vi "Database-ActorMain.vi"(0 "FTW Actor Instance Configuration":string="{\n  \"Identity\": \"ActorName\",\n  \"InboxAddress\": \"tcp://127.0.0.1:*\",\n  \"PublisherAddress\": \"tcp://127.0.0.1:*\",\n  \"DebugEnableInboxLogging\": false,\n  \"DebugEnableJobLogging\": false,\n  \"DebugShowPanel\": false\n}", 11 "error in":errorcluster) -> (15 "error out":errorcluster)   [LabVIEW 2013, in "PartCertDatabase-Actor.lvclass"]
uses:
  PartCertDatabase-Actor.lvclass
  ftw-dataflow/Actor/src/Instance/FTW-ActorInstance.lvclass
  ftw-dataflow/Actor/src/Message/Request/FTW-Message-IncomingRequest.lvclass
  PCert-Container/ERP-ConfigPageNewFeather/PCert-ConfigPageNF.lvclass
panel:
  # "Inputs"
  # "Outputs"
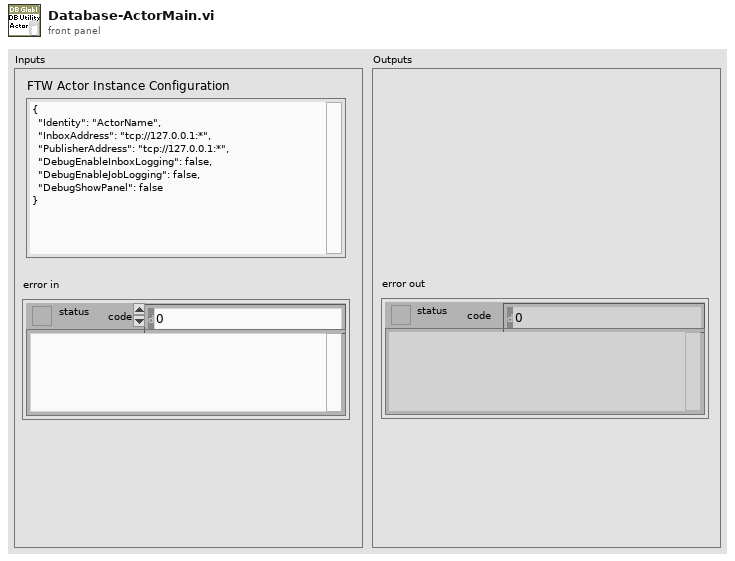
[diagram p1: front panel]
types:
  T1 = cluster{"Incoming Requests":refnum<event-registration>, "Additional Registration Types":refnum<event-registration>}
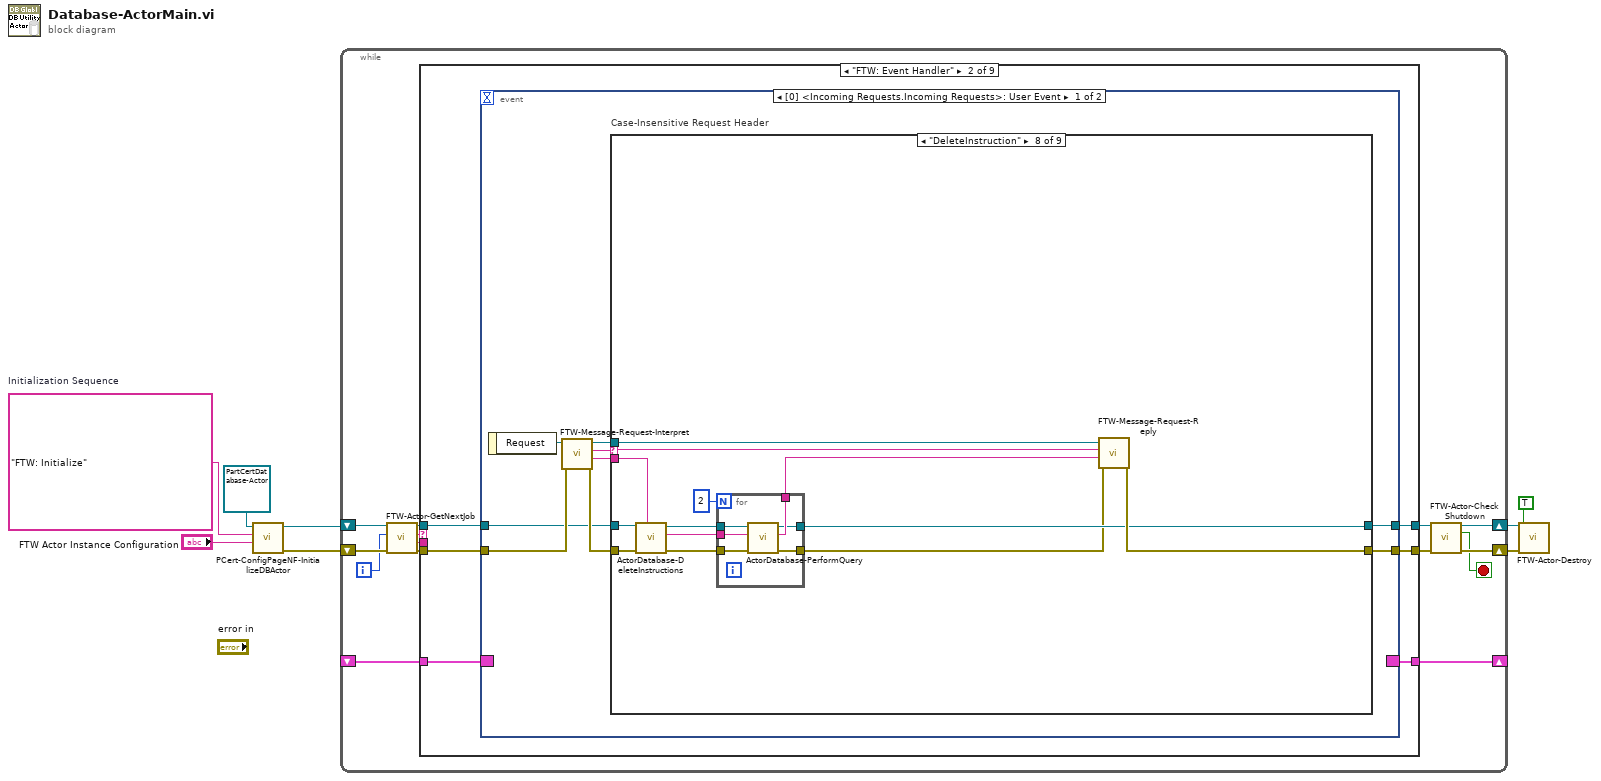
[diagram p0: block diagram]
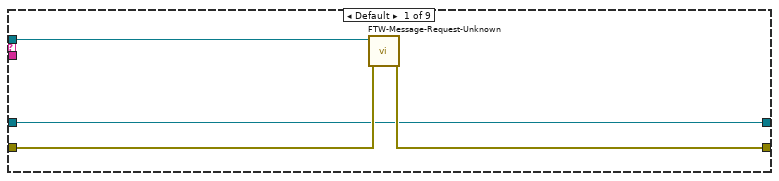
[diagram p3: hidden frame]
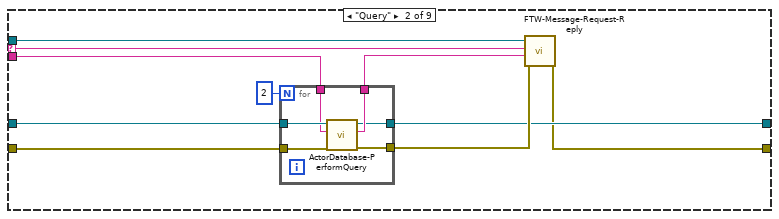
[diagram p4: hidden frame]
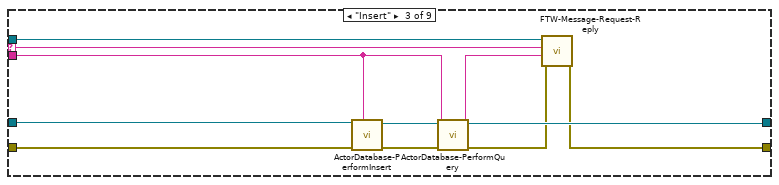
[diagram p5: hidden frame]
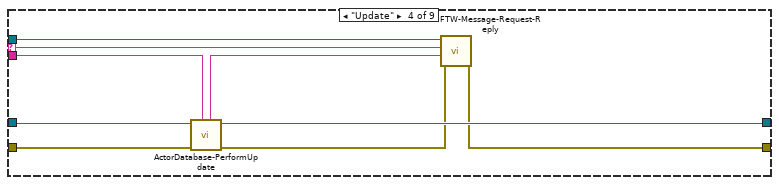
[diagram p6: hidden frame]
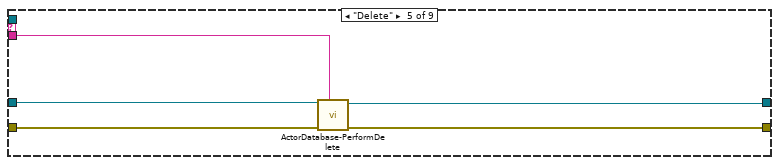
[diagram p7: hidden frame]
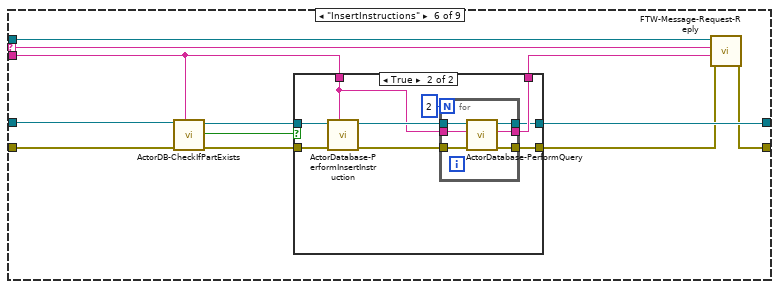
[diagram p8: hidden frame]
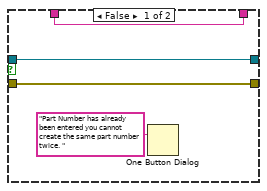
[diagram p9: hidden frame]
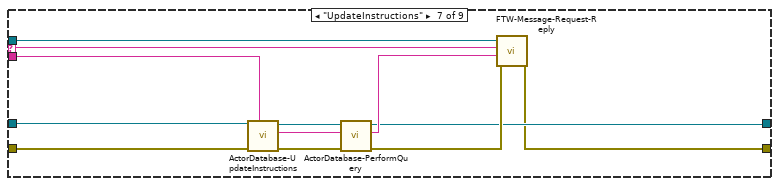
[diagram p10: hidden frame]
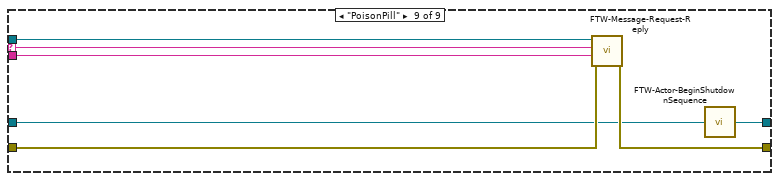
[diagram p11: hidden frame]
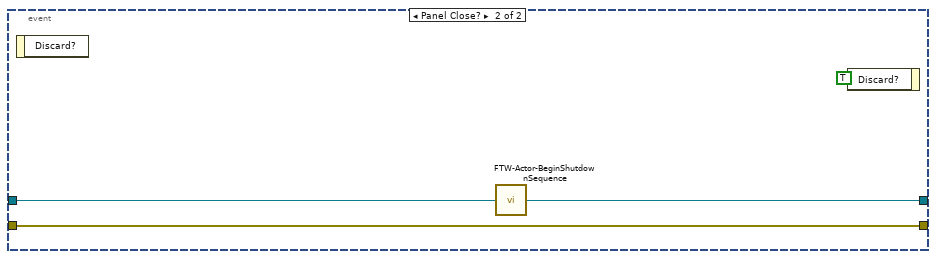
[diagram p12: hidden frame]
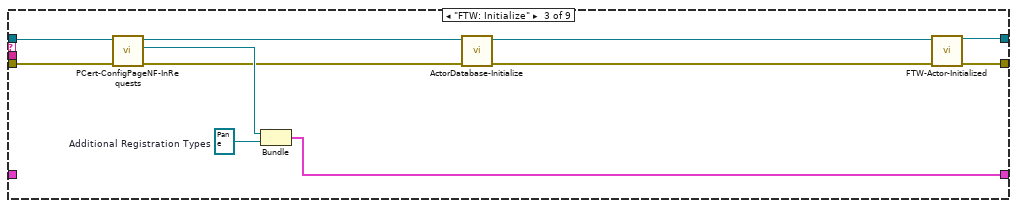
[diagram p13: hidden frame]
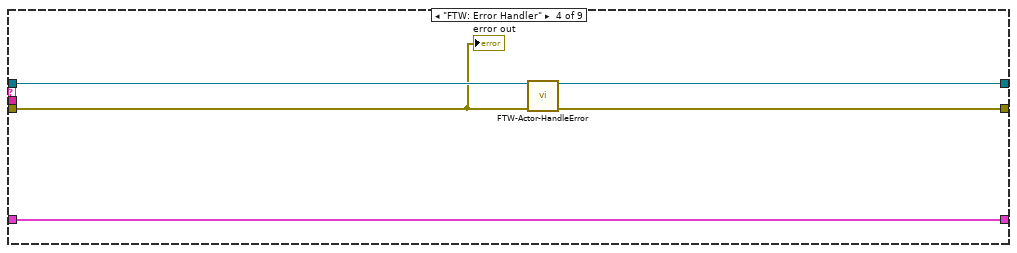
[diagram p14: hidden frame]
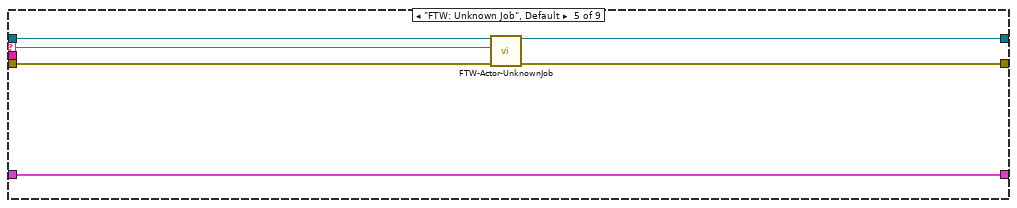
[diagram p15: hidden frame]
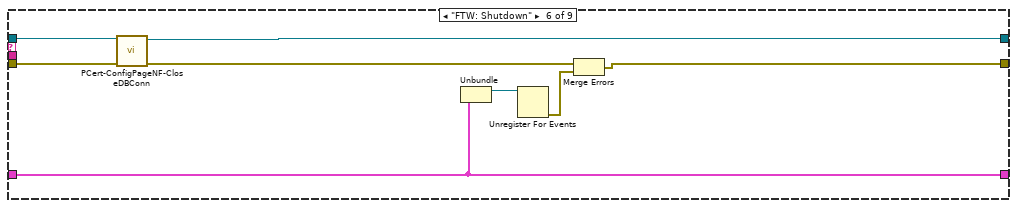
[diagram p16: hidden frame]
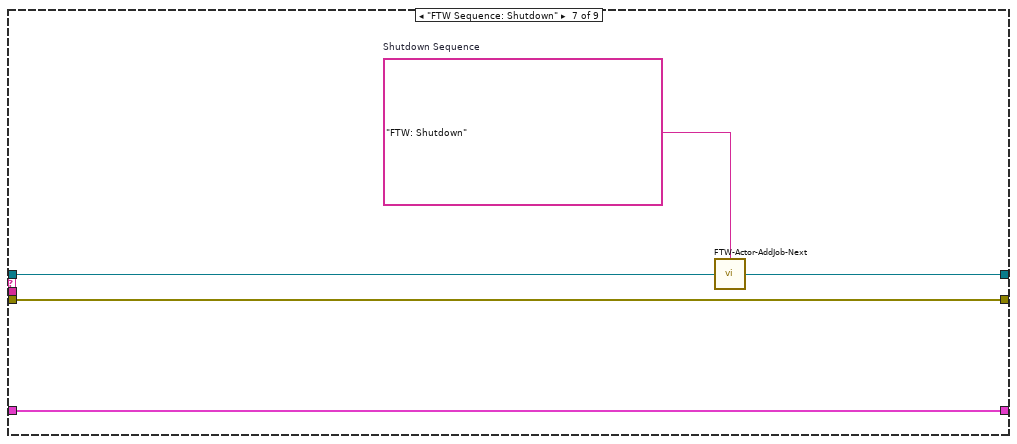
[diagram p17: hidden frame]
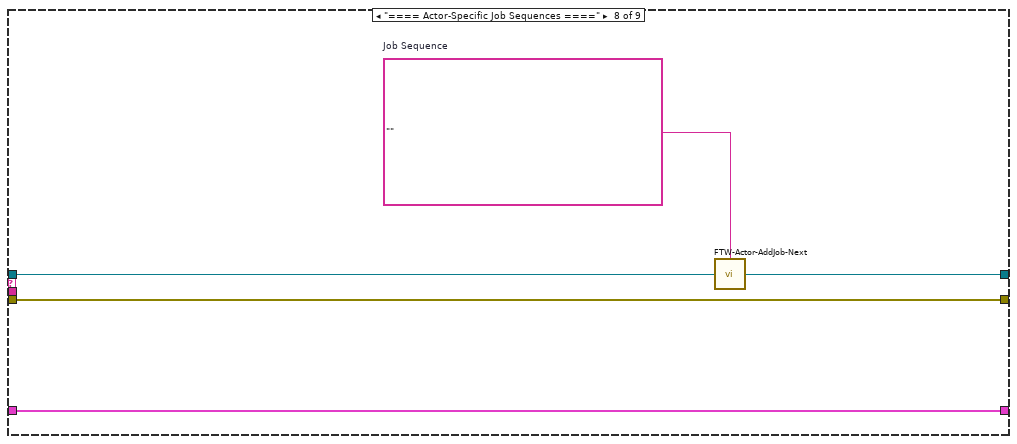
[diagram p18: hidden frame]
diagram:
  w4 = "FTW: Initialize"  # Initialization Sequence
  n1 = call-dynamic "PCert-ConfigPageNF-InitializeDBActor.vi"("FTW Actor Instance Configuration"="FTW Actor Instance Configuration", "Initialization Job Sequence"=w4, "ERP-ConfigPageNF.lvclass"=refnum<class "PartCertDatabase-Actor.lvclass"> refnum ("Database-Actor.lvclass")) -> ("error out"=w6:errorcluster, "ERP-ConfigPageNF out"=w3:refnum<class "PartCertDatabase-Actor.lvclass">)  [unwired: 7 in]
  n2 = while {
    shift-right: [w12] -> w7
    shift-left: w6 -> [w19]
    shift-right: [w9] -> _
    shift-left: _ -> [w22]
    shift-right: [w14] -> w8
    shift-left: w3 -> [w21]
    i -> [w10]
    stop <- w11 stop-if-true
    n3 = call "FTW-Actor-GetNextJob.vi"("error in"=w19, "Jobs Performed"=w10, "FTW Actor Instance"=w21) -> ("error out"=w18:errorcluster, "Job Data"=w16:string, "Job Name"=w17:string, "FTW Actor Instance out"=w20:refnum<class "PartCertDatabase-Actor.lvclass">)  [unwired: 5 in]
    n4 = case shown="\"FTW: Event Handler\"" w17 {
      selector: w17 -> [_ _ _ _ w175 _ _ _ _]
      tunnel: [w24 w31 w164 w171 w178 w186 w192 w197 w201] -> w13
      tunnel: w18 -> [w24 w30 w169 w170 w179 w183 w192 w197 w201]
      tunnel: w22 -> [w25 w26 _ w174 w180 w188 w193 w198 w200]
      tunnel: [w25 w29 w166 w174 w180 w188 w193 w198 w200] -> w9
      tunnel: w16 -> [_ _ _ _ _ _ _ _ _]
      tunnel: [w23 w28 w165 w172 w176 w182 w190 w195 w199] -> w15
      tunnel: w20 -> [w23 w27 w163 w173 w177 w184 w191 w196 w199]
      frame "==== Featherweight Framework Jobs ====" {
      }
      frame "FTW: Event Handler" {
        n5 = event shown="[0] <Incoming Requests.Incoming Requests>: User Event" {
          selector: w26 -> [_ _]
          dyn-events: [_ _] -> w29
          timeout: _ -> [_ _]
          tunnel: [w37 w157] -> w31
          tunnel: w30 -> [w38 w157]
          tunnel: [w36 w155] -> w28
          tunnel: w27 -> [w35 w156]
          event User Event {
            n6 = event-data() -> ("Request"=w39:refnum<class "FTW-Message-IncomingRequest.lvclass">)  [unwired: 1 in]
            n7 = call "FTW-Message-Request-Interpret.vi"("error in"=w38, "FTW Incoming Request"=w39) -> ("error out"=w40:errorcluster, "Request Body"=w33:string, "Request Header"=w34:string, "FTW Incoming Request out"=w32:refnum<class "FTW-Message-IncomingRequest.lvclass">)  [unwired: 6 in]
            n8 = case "Case-Insensitive Request Header" shown="\"DeleteInstruction\"" w34 {
              selector: w34 -> [_ w47 w66 w74 _ w92 w121 w138 w150]
              tunnel: [w43 w46 w63 w72 w83 w94 w118 w137 w151] -> w37
              tunnel: w40 -> [w44 w54 w62 w80 w85 w90 w128 w141 w152]
              tunnel: [w41 w48 w67 w77 w84 w96 w119 w133 w154] -> w36
              tunnel: w35 -> [w41 w53 w61 w79 w82 w91 w127 w140 w148]
              tunnel: w33 -> [_ w52 w69 w78 w81 w89 w124 w135 w149]
              tunnel: w32 -> [w42 w51 w68 w76 _ w93 w122 w139 w153]
              frame Default {
                n9 = call "FTW-Message-Request-Unknown.vi"("error in"=w44, "FTW Incoming Request"=w42) -> ("error out"=w43:errorcluster)  [unwired: 9 in]
              }
              frame "Query" {
                n10 = for {
                  N: 2 -> [_]
                  tunnel: w54 -> [w60]
                  tunnel: w53 -> [w59]
                  tunnel: w52 -> [w58]
                  tunnel: [w57] -> w50
                  tunnel: [w56] -> w49
                  tunnel: [w55] -> w48
                  n11 = call "ActorDatabase-PerformQuery.vi"("error in (no error)"=w60, "Payload from Actor"=w58, "Database-Actor in"=w59) -> ("error out"=w56:errorcluster, "Payload To Actor"=w57:string, "Database-Actor out"=w55:refnum<class "PartCertDatabase-Actor.lvclass">)  [unwired: 6 in]
                }
                n12 = call "FTW-Message-Request-Reply.vi"("error in"=w49, "Response Body"=w50, "Response Header"=w47, "FTW Incoming Request"=w51) -> ("error out"=w46:errorcluster)  [unwired: 6 in, 1 out]
              }
              frame "Insert" {
                n13 = call "ActorDatabase-PerformInsert.vi"("Payload From Actor"=w69, "error in (no error)"=w62, "Database-Actor in"=w61) -> ("error out"=w71:errorcluster, "Database-Actor out"=w70:refnum<class "PartCertDatabase-Actor.lvclass">)  [unwired: 7 in]
                n14 = call "ActorDatabase-PerformQuery.vi"("error in (no error)"=w71, "Payload from Actor"=w69, "Database-Actor in"=w70) -> ("error out"=w64:errorcluster, "Payload To Actor"=w65:string, "Database-Actor out"=w67:refnum<class "PartCertDatabase-Actor.lvclass">)  [unwired: 6 in]
                n15 = call "FTW-Message-Request-Reply.vi"("error in"=w64, "Response Body"=w65, "Response Header"=w66, "FTW Incoming Request"=w68) -> ("error out"=w63:errorcluster)  [unwired: 6 in, 1 out]
              }
              frame "Update" {
                n16 = call "ActorDatabase-PerformUpdate.vi"("Payload From Actor"=w78, "error in (no error)"=w80, "Database-Actor in"=w79) -> ("error out"=w73:errorcluster, "Database-Actor out"=w77:refnum<class "PartCertDatabase-Actor.lvclass">, "Payload to Actor"=w75:string)  [unwired: 6 in]
                n17 = call "FTW-Message-Request-Reply.vi"("error in"=w73, "Response Body"=w75, "Response Header"=w74, "FTW Incoming Request"=w76) -> ("error out"=w72:errorcluster)  [unwired: 6 in, 1 out]
              }
              frame "Delete" {
                n18 = call "ActorDatabase-PerformDelete.vi"("Payload From Actor"=w81, "error in (no error)"=w85, "Database-Actor in"=w82) -> ("error out"=w83:errorcluster, "Database-Actor out"=w84:refnum<class "PartCertDatabase-Actor.lvclass">)  [unwired: 7 in]
              }
              frame "InsertInstructions" {
                n19 = call "ActorDB-CheckIfPartExists.vi"("Request Body"=w89, "error in"=w90, "Database-Actor in"=w91) -> ("error out"=w88:errorcluster, "Part number not found?"=w86:bool, "Database-Actor out"=w87:refnum<class "PartCertDatabase-Actor.lvclass">)  [unwired: 6 in]
                n20 = case shown="True" w86 {
                  tunnel: [w101 w109] -> w97
                  tunnel: [w100 w108] -> w96
                  tunnel: [w99 w107] -> w95
                  tunnel: w89 -> [w101 w106]
                  tunnel: w88 -> [w99 w105]
                  tunnel: w87 -> [w100 w104]
                  frame False {
                    n21 = One Button Dialog(message="Part Number has already been entered you cannot create the same part number twice. ") -> ()  [unwired: 1 in, 1 out]
                  }
                  frame True {
                    n22 = call "ActorDatabase-PerformInsertInstruction.vi"("Payload From Actor"=w106, "error in (no error)"=w105, "Database-Actor in"=w104) -> ("error out"=w102:errorcluster, "Database-Actor out"=w110:refnum<class "PartCertDatabase-Actor.lvclass">)  [unwired: 7 in]
                    n23 = for {
                      N: 2 -> [_]
                      tunnel: w110 -> [w116]
                      tunnel: [w115] -> w109
                      tunnel: [w114] -> w108
                      tunnel: [w113] -> w107
                      tunnel: w106 -> [w112]
                      tunnel: w102 -> [w111]
                      n24 = call "ActorDatabase-PerformQuery.vi"("error in (no error)"=w111, "Payload from Actor"=w112, "Database-Actor in"=w116) -> ("error out"=w113:errorcluster, "Payload To Actor"=w115:string, "Database-Actor out"=w114:refnum<class "PartCertDatabase-Actor.lvclass">)  [unwired: 6 in]
                    }
                  }
                }
                n25 = call "FTW-Message-Request-Reply.vi"("error in"=w95, "Response Body"=w97, "Response Header"=w92, "FTW Incoming Request"=w93) -> ("error out"=w94:errorcluster)  [unwired: 6 in, 1 out]
              }
              frame "UpdateInstructions" {
                n26 = call "ActorDatabase-UpdateInstructions.vi"("Payload From Actor"=w124, "error in (no error)"=w128, "Database-Actor in"=w127) -> ("error out"=w126:errorcluster, "JSON Query"=w117:string, "Database-Actor out"=w125:refnum<class "PartCertDatabase-Actor.lvclass">)  [unwired: 6 in]
                n27 = call "ActorDatabase-PerformQuery.vi"("error in (no error)"=w126, "Payload from Actor"=w117, "Database-Actor in"=w125) -> ("error out"=w120:errorcluster, "Payload To Actor"=w123:string, "Database-Actor out"=w119:refnum<class "PartCertDatabase-Actor.lvclass">)  [unwired: 6 in]
                n28 = call "FTW-Message-Request-Reply.vi"("error in"=w120, "Response Body"=w123, "Response Header"=w121, "FTW Incoming Request"=w122) -> ("error out"=w118:errorcluster)  [unwired: 6 in, 1 out]
              }
              frame "DeleteInstruction" {
                n29 = call "ActorDatabase-DeleteInstructions.vi"("Payload From Actor"=w135, "error in (no error)"=w141, "Database-Actor in"=w140) -> ("error out"=w130:errorcluster, "New Payload"=w131:string, "Database-Actor out"=w136:refnum<class "PartCertDatabase-Actor.lvclass">)  [unwired: 6 in]
                n30 = for {
                  N: 2 -> [_]
                  tunnel: w136 -> [w147]
                  tunnel: [w146] -> w134
                  tunnel: [w145] -> w133
                  tunnel: [w144] -> w132
                  tunnel: w131 -> [w143]
                  tunnel: w130 -> [w142]
                  n31 = call "ActorDatabase-PerformQuery.vi"("error in (no error)"=w142, "Payload from Actor"=w143, "Database-Actor in"=w147) -> ("error out"=w144:errorcluster, "Payload To Actor"=w146:string, "Database-Actor out"=w145:refnum<class "PartCertDatabase-Actor.lvclass">)  [unwired: 6 in]
                }
                n32 = call "FTW-Message-Request-Reply.vi"("error in"=w132, "Response Body"=w134, "Response Header"=w138, "FTW Incoming Request"=w139) -> ("error out"=w137:errorcluster)  [unwired: 6 in, 1 out]
              }
              frame "PoisonPill" {
                n33 = call "FTW-Message-Request-Reply.vi"("error in"=w152, "Response Body"=w149, "Response Header"=w150, "FTW Incoming Request"=w153) -> ("error out"=w151:errorcluster)  [unwired: 6 in, 1 out]
                n34 = call "FTW-Actor-BeginShutdownSequence.vi"("FTW Actor Instance"=w148) -> ("FTW Actor Instance out"=w154:refnum<class "PartCertDatabase-Actor.lvclass">)  [unwired: 3 in]
              }
            }
          }
          event Panel Close? {
            n35 = event-data() -> ()  [unwired: 1 in, 1 out]
            n36 = call "FTW-Actor-BeginShutdownSequence.vi"("FTW Actor Instance"=w156) -> ("FTW Actor Instance out"=w155:refnum<class "PartCertDatabase-Actor.lvclass">)  [unwired: 3 in]
            n37 = event-data("Discard?"=TRUE) -> ()  [unwired: 1 in, 1 out]
          }
        }
      }
      frame "FTW: Initialize" {
        w168 = refnum<event-registration> refnum  # Additional Registration Types
        n38 = call "PCert-ConfigPageNF-InRequests.vi"("error in (no error)"=w169, "ERP-ConfigPageNF in"=w163) -> ("error out"=w162:errorcluster, "Incoming Requests"=w167:refnum<event-registration>, "ERP-ConfigPageNF out"=w161:refnum<class "PartCertDatabase-Actor.lvclass">)  [unwired: 7 in]
        n39 = Bundle("Incoming Requests"=w167, "Additional Registration Types"=w168) -> (w166:T1)  [unwired: 1 in]
        n40 = call "ActorDatabase-Initialize.vi"("error in (no error)"=w162, "Database-Actor In"=w161) -> ("error out"=w159:errorcluster, "Database-Actor out"=w160:refnum<class "PartCertDatabase-Actor.lvclass">)  [unwired: 8 in]
        n41 = call-dynamic "FTW-Actor-Initialized.vi"("FTW Actor Instance"=w160, "error in"=w159) -> ("FTW Actor Instance out"=w165:refnum<class "PartCertDatabase-Actor.lvclass">, "error out"=w164:errorcluster)  [unwired: 12 in]
      }
      frame "FTW: Error Handler" {
        n42 = call-dynamic "FTW-Actor-HandleError.vi"("FTW Actor Instance"=w173, "error in"=w170) -> ("FTW Actor Instance out"=w172:refnum<class "PartCertDatabase-Actor.lvclass">, "error out"=w171:errorcluster)  [unwired: 11 in, 1 out]
        "error out" <- w170
      }
      frame "FTW: Unknown Job", Default {
        n43 = call-dynamic "FTW-Actor-UnknownJob.vi"("FTW Actor Instance"=w177, "Unknown Job"=w175, "error in"=w179) -> ("FTW Actor Instance out"=w176:refnum<class "PartCertDatabase-Actor.lvclass">, "error out"=w178:errorcluster)  [unwired: 11 in]
      }
      frame "FTW: Shutdown" {
        n44 = call "PCert-ConfigPageNF-CloseDBConn.vi"("error in (no error)"=w183, "ERP-ConfigPageNF in"=w184) -> ("error out"=w181:errorcluster, "ERP-ConfigPageNF out"=w182:refnum<class "PartCertDatabase-Actor.lvclass">)  [unwired: 8 in]
        n45 = Unbundle(w188) -> ("Incoming Requests"=w187:refnum<event-registration>)  [unwired: 1 out]
        n46 = Unregister For Events(event registration refnum=w187) -> (error out=w185:errorcluster)  [unwired: 1 in]
        n47 = Merge Errors(w181, w185) -> (w186:errorcluster)
      }
      frame "FTW Sequence: Shutdown" {
        w189 = "FTW: Shutdown"  # Shutdown Sequence
        n48 = call "FTW-Actor-AddJob-Next.vi"("Add Next in Job Queue"=w189, "FTW Actor Instance"=w191) -> ("FTW Actor Instance out"=w190:refnum<class "PartCertDatabase-Actor.lvclass">)  [unwired: 2 in]
      }
      frame "==== Actor-Specific Job Sequences ====" {
        w194 = ""  # Job Sequence
        n49 = call "FTW-Actor-AddJob-Next.vi"("Add Next in Job Queue"=w194, "FTW Actor Instance"=w196) -> ("FTW Actor Instance out"=w195:refnum<class "PartCertDatabase-Actor.lvclass">)  [unwired: 2 in]
      }
      frame "==== Actor-Specific Jobs ====" {
      }
    }
    n50 = call "FTW-Actor-CheckShutdown.vi"("FTW Actor Instance"=w15, "error in"=w13) -> ("FTW Actor Instance out"=w14:refnum<class "PartCertDatabase-Actor.lvclass">, "Shutdown?"=w11:bool, "error out"=w12:errorcluster)  [unwired: 11 in]
  }
  n51 = call-dynamic "FTW-Actor-Destroy.vi"("FTW Actor Instance"=w8, "Force Destroy?"=TRUE, "error in"=w7) -> ()  [unwired: 12 in, 1 out]
